vi "MGI SZL Zip Directory.vi"(4 "Folders to Exclude":string[](array[string]), 6 "updateMode (Safe)":i32(ring) items=["Safe", "Direct"], 7 "Open Options (Create New)":T1, 8 "Error In":errorcluster, 9 "Include Subdirectories? (F)":bool, 10 "Zip File":path=path "D:/BigZip", 11 "Root Directory":path=path "D:/Depot") -> (0 "Error Out":errorcluster, 2 "Zip File Out":path, 3 "Root Directory Out":path)   [LabVIEW 2020]
doc: "Compresses everything in root directory into a zip file. If include subdirectories? is TRUE, this VI recursively includes any subdirectories. Open Options can be set to create the zip file new, or open an existing one and append on to it.\n\nThis VI relies on the Sharp Zip Library which is a .NET assembly written in C# by Mike Krueger. It is licenced under the GPL with a special exception permitting independent modules to link to the library regardless of the license terms of the independent module. \n\nMore information about the library and its license is available from:\nhttp://www.icsharpcode.net/opensource/sharpziplib/"
uses:
  <userlib>/_MGI/File/Zip/MGI SZL Open Options.ctl
  C:/Program Files/National Instruments/LabVIEW 2020/user.lib/_MGI/File/Zip/Support Files/ICSharpCode.SharpZipLib.dll
  Support Files/ICSharpCode.SharpZipLib.dll
panel:
  out "Elapsed Time (msec)":u32
  out "Progress":i32(slide) scale=0.0..2.0
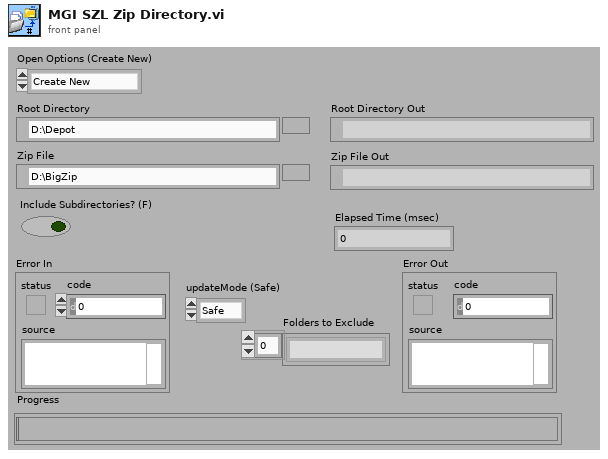
[diagram p1: front panel]
types:
  T1 = typedef "MGI SZL Open Options.ctl" = enum16{"Create New", "Append To Existing"}
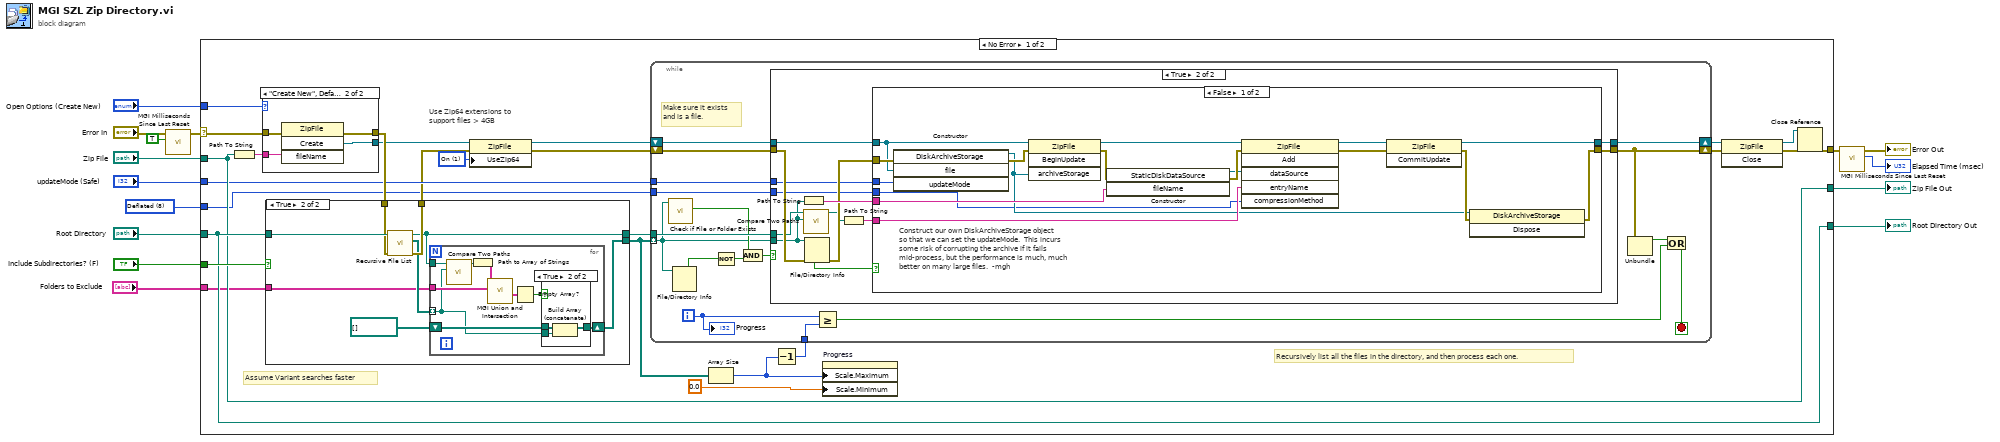
[diagram p0: block diagram]
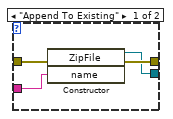
[diagram p4: hidden frame]
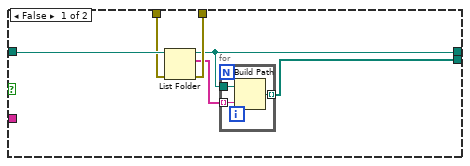
[diagram p5: hidden frame]
diagram:
  w2 = 8 items=["Stored"=0, "Deflated"=8, "Deflate64"=9, "BZip2"=11, "WinZipAES"=99] ("compressionMethod (Deflated)")
  n1 = call <userlib>:"MGI Milliseconds Since Last Reset.vi"("Reset (F)"=TRUE ("Reset"), "Error In"="Error In") -> ("Error Out"=w7:errorcluster)  [unwired: 4 in, 1 out]
  n2 = case shown="No Error" w7 {
    selector: w7 -> [w30 w132]
    tunnel: [w35 w132] -> w5
    tunnel: "Include Subdirectories? (F)" -> [w34 _]
    tunnel: "Open Options (Create New)" -> [w33 _]
    tunnel: "Zip File" -> [w31 w131]
    tunnel: "Root Directory" -> [w32 w130]
    tunnel: [w32 w130] -> w11
    tunnel: [w31 w131] -> w10
    tunnel: "updateMode (Safe)" -> [w23 _]
    tunnel: w2 -> [w17 _]
    tunnel: "Folders to Exclude" -> [w16 _]
    frame No Error {
      w18 = 1 items=["Off", "On", "Dynamic"] ("UseZip64")
      # "Assume Variant searches faster"
      # "Use Zip64 extensions to\nsupport files > 4GB"
      # "Recursively list all the files in the directory, and then process each one."
      n3 = Path To String(path=w31) -> (string=w37:string)
      n4 = case shown="\"Create New\", Default" w33 {
        tunnel: w37 -> [w93 w99]
        tunnel: [w92 w98] -> w22
        tunnel: [w95 w97] -> w36
        tunnel: w30 -> [w94 w96]
        frame "Append To Existing" {
          n5 = constructor class="ZipFile"(error in=w94, "name"=w93) -> (reference out=w92:refnum<k24>, error out=w95:errorcluster)  [unwired: 2 in, 2 out]
        }
        frame "Create New", Default {
          n6 = invoke class="ZipFile" method="Create"(error in=w96, "fileName"=w99) -> (error out=w97:errorcluster, "Create"=w98:refnum<k24>)  [unwired: 2 in, 2 out]
        }
      }
      n7 = case shown="True" w34 {
        tunnel: w32 -> [w105 w116]
        tunnel: [w103 w115] -> w20
        tunnel: [w100 w109] -> w28
        tunnel: [w101 w112] -> w38
        tunnel: w36 -> [w104 w114]
        tunnel: w16 -> [_ w111]
        frame False {
          n8 = List Folder(path=w105, error in=w104) -> (path out=w101:path, filenames=w102:string[], error out=w103:errorcluster)  [unwired: 2 in, 1 out]
          n9 = for {
            tunnel: w102 -> [w108] mode=indexing
            tunnel: w101 -> [w107]
            tunnel: [w106] -> w100 mode=indexing
            n10 = Build Path(base path=w107, name or relative path=w108) -> (appended path=w106:path)
          }
        }
        frame True {
          n11 = call <vilib>:"Recursive File List.vi"("error in (no error)"=w114, "Folder Path"=w116) -> ("error out"=w115:errorcluster, "All Files in Dir"=w113:path[], "dup Folder Path"=w112:path)  [unwired: 5 in, 2 out]
          n12 = for {
            tunnel: w113 -> [w118] mode=indexing
            tunnel: w112 -> [w125]
            tunnel: w111 -> [w123]
            shift-right: [w117] -> w109
            shift-left: path[] [] ("All Files in Dir") -> [w119]
            n13 = call <vilib>:"Compare Two Paths.vi"("Path 2"=w118, "Path 1"=w125) -> ("Relative Path from 1 to 2"=w124:path)  [unwired: 6 in, 3 out]
            n14 = Path to Array of Strings(0:w124) -> (2:w122:string[])  [unwired: 1 out]
            n15 = call <userlib>:"MGI Union and Intersection.vi"("Sequence 2[]"=w123, "Sequence 1[]"=w122) -> ("Intersection[]"=w121:string[])  [unwired: 6 in, 3 out]
            n16 = Empty Array?(array=w121) -> (empty?=w120:bool)
            n17 = case shown="True" w120 {
              tunnel: w119 -> [w126 w129]
              tunnel: w118 -> [_ w128]
              tunnel: [w126 w127] -> w117
              frame False {
              }
              frame True {
                n18 = Build Array (concatenate)(w129, w128) -> (w127:path[])
              }
            }
          }
        }
      }
      n19 = property class="ZipFile"(reference=w22, error in=w20, "UseZip64"=w18) -> (reference out=w21:refnum<k24>, error out=w19:errorcluster)
      n20 = Array Size(array=w28) -> (size(s)=w25:i32)
      n21 = Decrement(x=w25) -> (x-1=w24:i32)
      n22 = while {
        shift-right: [w50] -> w26
        shift-left: w19 -> [w46]
        tunnel: w28 -> [w41] mode=indexing
        tunnel: w38 -> [w56]
        shift-right: [w57] -> w27
        shift-left: w21 -> [w47]
        tunnel: w24 -> [w52]
        tunnel: w23 -> [w45]
        tunnel: w17 -> [w44]
        i -> [w53]
        stop <- w49 stop-if-true
        # "Make sure it exists\nand is a file."
        n23 = call <vilib>:"Check if File or Folder Exists.vi"("path"=w41) -> ("file or folder exists?"=w43:bool)  [unwired: 8 in, 2 out]
        n24 = File/Directory Info(path=w41) -> (directory=w42:bool)  [unwired: 1 in, 6 out]
        n25 = Not(x=w42) -> (.not. x?=w54:bool)
        n26 = And(x=w43, y=w54) -> (x .and. y?=w55:bool)
        n27 = case shown="True" w55 {
          tunnel: w47 -> [w59 w67]
          tunnel: [w59 w71] -> w57
          tunnel: w56 -> [_ w62]
          tunnel: w46 -> [w58 w66]
          tunnel: w41 -> [_ w61]
          tunnel: [w58 w64] -> w50
          tunnel: w45 -> [_ w65]
          tunnel: w44 -> [_ w63]
          frame False {
          }
          frame True {
            n28 = Path To String(path=w61) -> (string=w72:string)
            n29 = call <vilib>:"Compare Two Paths.vi"("Path 2"=w61, "Path 1"=w62) -> ("Relative Path from 1 to 2"=w60:path)  [unwired: 6 in, 3 out]
            n30 = File/Directory Info(path=w61, error in=w66) -> (error out=w68:errorcluster, shortcut=w69:bool)  [unwired: 5 out]
            n31 = Path To String(path=w60) -> (string=w70:string)
            n32 = case shown="False" w69 {
              tunnel: w72 -> [w78 _]
              tunnel: w67 -> [w86 w90]
              tunnel: [w89 w90] -> w71
              tunnel: [w83 w91] -> w64
              tunnel: w70 -> [w82 _]
              tunnel: w68 -> [w88 w91]
              tunnel: w65 -> [w85 _]
              tunnel: w63 -> [w74 _]
              frame False {
                # "Construct our own DiskArchiveStorage object\nso that we can set the updateMode.  This incurs\nsome risk of corrupting the archive if it fails\nmid-process, but the performance is much, much\nbetter on many large files.  -mgh"
                n33 = constructor class="DiskArchiveStorage"(error in=w88, "file"=w86, "updateMode"=w85) -> (reference out=w75:refnum<k24>, error out=w87:errorcluster)  [unwired: 2 in, 3 out]
                n34 = invoke class="ZipFile" method="BeginUpdate"(reference=w86, error in=w87, "archiveStorage"=w75) -> (reference out=w73:refnum<k24>, error out=w81:errorcluster)  [unwired: 1 in, 2 out]
                n35 = constructor class="StaticDiskDataSource"(error in=w81, "fileName"=w78) -> (reference out=w79:refnum<k24>, error out=w80:errorcluster)  [unwired: 2 in, 2 out]
                n36 = invoke class="ZipFile" method="Add"(reference=w73, error in=w80, "dataSource"=w79, "entryName"=w82, "compressionMethod"=w74) -> (reference out=w76:refnum<k24>, error out=w77:errorcluster)  [unwired: 1 in, 4 out]
                n37 = invoke class="ZipFile" method="CommitUpdate"(reference=w76, error in=w77) -> (reference out=w89:refnum<k24>, error out=w84:errorcluster)  [unwired: 1 in, 1 out]
                n38 = invoke class="DiskArchiveStorage" method="Dispose"(reference=w75, error in=w84) -> (error out=w83:errorcluster)  [unwired: 1 in, 2 out]
              }
              frame True {
                # "Don't archive shortcuts."
              }
            }
          }
        }
        n39 = Greater Or Equal?(x=w53, y=w52) -> (x >= y?=w48:bool)
        n40 = Unbundle(w50) -> ("status"=w51:bool)  [unwired: 2 out]
        n41 = Compound Arithmetic op=OR(w51, w48) -> (w49:bool)
        "Progress" <- w53
      }
      n42 = property on="Progress" class="Slide (strict)"("Scale.Maximum"=w25, "Scale.Minimum"=0.0 ("Scale.Range:Minimum")) -> ()  [unwired: 2 in, 2 out]
      n43 = invoke class="ZipFile" method="Close"(reference=w27, error in=w26) -> (reference out=w39:refnum<k24>, error out=w40:errorcluster)  [unwired: 1 in, 1 out]
      n44 = Close Reference(reference=w39, error in (no error)=w40) -> (error out=w35:errorcluster)
    }
    frame Error {
    }
  }
  "Zip File Out" <- w10
  "Root Directory Out" <- w11
  n45 = call <userlib>:"MGI Milliseconds Since Last Reset.vi"("Error In"=w5) -> ("ms"=→"Elapsed Time (msec)":u32, "Error Out"=→"Error Out":errorcluster)  [unwired: 5 in]
